vi "Sys config window-Get set control values.vi"(8 "error in (no error)":errorcluster, 11 "Function":T31) -> (0 "error out":errorcluster, 3 "output cluster":T1={"Triggers output setup"=[], "General trigger settings"={"Trigger 1 function"=enum."Encoder trigger", "Triggers loop clock (MHz)"=80.0}, "Calibration settings"={"Pockels cal.Zoom"=0, "Pockels cal.Dwell time (µs)"=0.0}, "Hardware Configuration"={"Dev. PC"=FALSE, "Swap XY on stage"=FALSE, "No of AOD"=0, "Computer MAC address"="", "Externalise Triggers"=FALSE, "Trigger HW config"={"Available Device List"=0, "Device Address"=""}, "DAQmx Chan"={"Pockels AO"="", "Hard shutter AO"="", "PMT AOs"="", "Galvo AOs"="", "Power meter AI"=""}, "XY stage available"=FALSE, "XY Stage"={"COM port"="", "Baudrate"=0, "Type"=""}, "Z stage available"=FALSE, "Z Stage config cluster"={"COM port"="COM7", "Baudrate"=0, "Type"=""}, "Encoder available"=FALSE, "Encoder"={"IP address"="224.0.1.103", "Port"=7000, "Wheel radius (cm)"=16.0, "Encoder Trigger"=""}, "VidRec available"=FALSE, "Cam VidRec"={"DO flag-Video record"="", "DO flag-Trial start"=""}, "Laser Power Control HW config"={"Laser Power Control"="", "Laser Power Modulation Control"=enum."NI"}, "Laser 1 available"=FALSE, "Laser 1 config cluster"={"COM port"="COM7", "Baud Rate"=0, "Type"=""}, "Prechirper 1 available"=FALSE, "Prechirper 1 config cluster"={"Type"="", "Baud Rate"=0, "COM port"="COM7"}, "Control system.FPGA available?"=FALSE, "Control Sys. HW config"={"Control system.FPGA Type"=enum."Virtex 5", "Control system.Network adapter name"="", "Control system.MAC address"="", "Control system.Ethernet Port"=0, "Control system.Ethernet Port Opened"=FALSE}, "DAQ FPGA HW Config"={"FGPA Ref"=refnum, "Target"="RIO0", "input card type"=enum."AC Card"}}, "System Config"={"Laser wavelength (nm)"=920.0, "DAQ FPGA System"={"Clock Freq (MHz) "=200.0, "Samples Wait after Trigger"=5080, "AOD fill"=4900, "StartupDelay"=0, "Slip Cycle (clock cycles)"=600000, "Add Cycle"=TRUE}, "Control system"={"AOD 1 Amplitude"=0, "AOD 2 Amplitude"=0, "AOD 3 Amplitude"=0, "AOD 4 Amplitude"=0, "AOD 5 Amplitude"=0, "AOD 6 Amplitude"=0, "T0 (ns)"=0.0, "Ta (ns)"=0.0, "Data Time Interval (ns)"=0.0, "Ctrl FPGA Clock (MHz)"=240.0}}, "Calibration config."={"Current Objective"="", "Objective Settings"=[], "PreChirper Values Preset ?"=FALSE, "PreChirper Settings"=[], "PreChirper Constants"={"a 1"=0, "b 1"=0, "c 1"=0, "a 2"=0, "b 2"=0, "c 2"=0, "lmin"=0, "lmax"=0}}, "General Setup"={"Microscope ID"="003", "Microscope Type"="AOLM", "Revision Number"="1.0.0.0", "Advanced Imaging"=FALSE, "Error Logging"=FALSE, "Performance Monitoring"=FALSE, "Max Allowed Trial Length"=60.0, "Initial Scan Resolution"=512.0, "Initial Acceptance Angle"=5.0, "Initial Laser Wavelength"=900.0, "Initial Dwell Time"=900.0}, "AOD Settings - distilled"={"AOD 1 thickness (mm)"=8.0, "AOD 2 thickness (mm)"=8.0, "AOD 3 thickness (mm)"=8.0, "AOD 4 thickness (mm)"=8.0, "AOD 1-2 separation (mm)"=50.0, "AOD 2-3 separation (mm)"=50.0, "AOD 3-4 separation (mm)"=50.0, "AOD 1 Centre (mm)"=7.5, "AOD 2 Centre (mm)"=7.5, "AOD 3 Centre (mm)"=7.5, "AOD 4 Centre (mm)"=7.5, "AOD 1 X Offset"=0.0, "AOD 2 X Offset"=0.0023, "AOD 3 X Offset"=0.0046, "AOD 4 X Offset"=0.0046, "AOD 1 Y Offset"=0.0, "AOD 2 Y Offset"=0.0, "AOD 3 Y Offset"=0.0023, "AOD 4 Y Offset"=0.0046, "Timing Offset AOD 1"=0.0, "Timing Offset AOD 2"=0.0, "Timing Offset AOD 3"=0.0, "Timing Offset AOD 4"=0.0, "AOL centre wavelength (nm)"=1.0, "AOL centre frequency (MHz)"=1.0, "Pair deflection ratio"=1.0, "AOL aperture (mm)"=15.0, "AOD fill time (us)"=1.0, "Diffraction mode"=1.0, "Crystal length (mm)"=0.0, "Acoustic velocity (m/s)"=1.0, "AOD Ord. Refractive index"=2.22}} {"System Config"."Control system"."Ctrl FPGA Clock (MHz)" min=80.0 max=500.0 step=1.0; "System Config"."Control system"."Data Time Interval (ns)" min=0.0 max=2048.0 step=1.0; "System Config"."Control system"."Ta (ns)" min=0.0 max=2048.0 step=1.0; "System Config"."Control system"."T0 (ns)" min=0.0 max=2048.0 step=1.0; "System Config"."Control system"."AOD 6 Amplitude" min=0 max=2048 step=1; "System Config"."Control system"."AOD 5 Amplitude" min=0 max=2048 step=1; "System Config"."Control system"."AOD 4 Amplitude" min=0 max=2048 step=1; "System Config"."Control system"."AOD 3 Amplitude" min=0 max=2048 step=1; "System Config"."Control system"."AOD 2 Amplitude" min=0 max=2048 step=1; "System Config"."Control system"."AOD 1 Amplitude" min=0 max=2048 step=1; "System Config"."Laser wavelength (nm)" min=800.0 max=1080.0 step=1.0; "Hardware Configuration"."Encoder"."Wheel radius (cm)" format="%#_13g"; "General trigger settings"."Triggers loop clock (MHz)" format="%#_13g"; "Triggers output setup"."Pulse width (us)" min=10 max=5000 step=1 format="%.0fµs"})   [LabVIEW 2017]
uses:
  Visualisation/Functional Imaging Viewer/Typedefs/Get-Set-Clear Control.ctl
  Configuration code/Typedefs/Initial config.ctl
  Peripherals Control/Triggers/Typedefs/Triggers output setup.ctl
  Peripherals Control/Triggers/Typedefs/Trigger setup element cluster.ctl
  Peripherals Control/Triggers/Typedefs/General trigger settings cluster.ctl
  Typedefs/Trigger 1 selector enum.ctl
  Configuration code/Typedefs/Pockels Calibration settings cluster.ctl
  Typedefs/Hardware Configuration settings.ctl
  Typedefs/Triggers HW config.ctl
  Typedefs/DAQmx physical channels cluster.ctl
  Typedefs/XY Stage config cluster.ctl
  Typedefs/Z Stage config cluster.ctl
  Typedefs/Encoder config cluster.ctl
  Typedefs/Cam VidRec HW config setup cluster.ctl
  Typedefs/Laser Power Control HW config.ctl
  Typedefs/Laser 1 config cluster.ctl
  Typedefs/PreChirper 1 config cluster.ctl
  Typedefs/Control Sys HW config cluster.ctl
  Typedefs/DAQ FPGA HW config cluster.ctl
  RIG-SPECIFIC FILES/FPGA Refs/FPGA Ref.ctl
  <vilib>/userdefined/High Color/nirio_resource_hc.ctl
  Typedefs/FPGA input type AC-DC.ctl
  Typedefs/System Configuration.ctl
  Typedefs/DAQ FPGA system config.ctl
  Typedefs/CTRL system config.ctl
  Typedefs/Calibration config.ctl
  Typedefs/Objective Config.ctl
  Typedefs/Prechirper Cal Config.ctl
  Typedefs/PreChirper constants.ctl
  Typedefs/General Setup.ctl
  Typedefs/AOD Settings-distilled.ctl
  Typedefs/HW config states enum.ctl
  Typedefs/fgv_actions.ctl
  Globals/Sys Config window globals.vi
  Global Variables/General Globals.vi
  Configuration code/Calibration/Globals/gl_Calibration globals.vi
panel:
  # "Thickness (mm)"
  # "X Offset"
  # "Separation (mm)"
  # "Y Offset"
  # "Centre (mm)"
  # "Timing Offset"
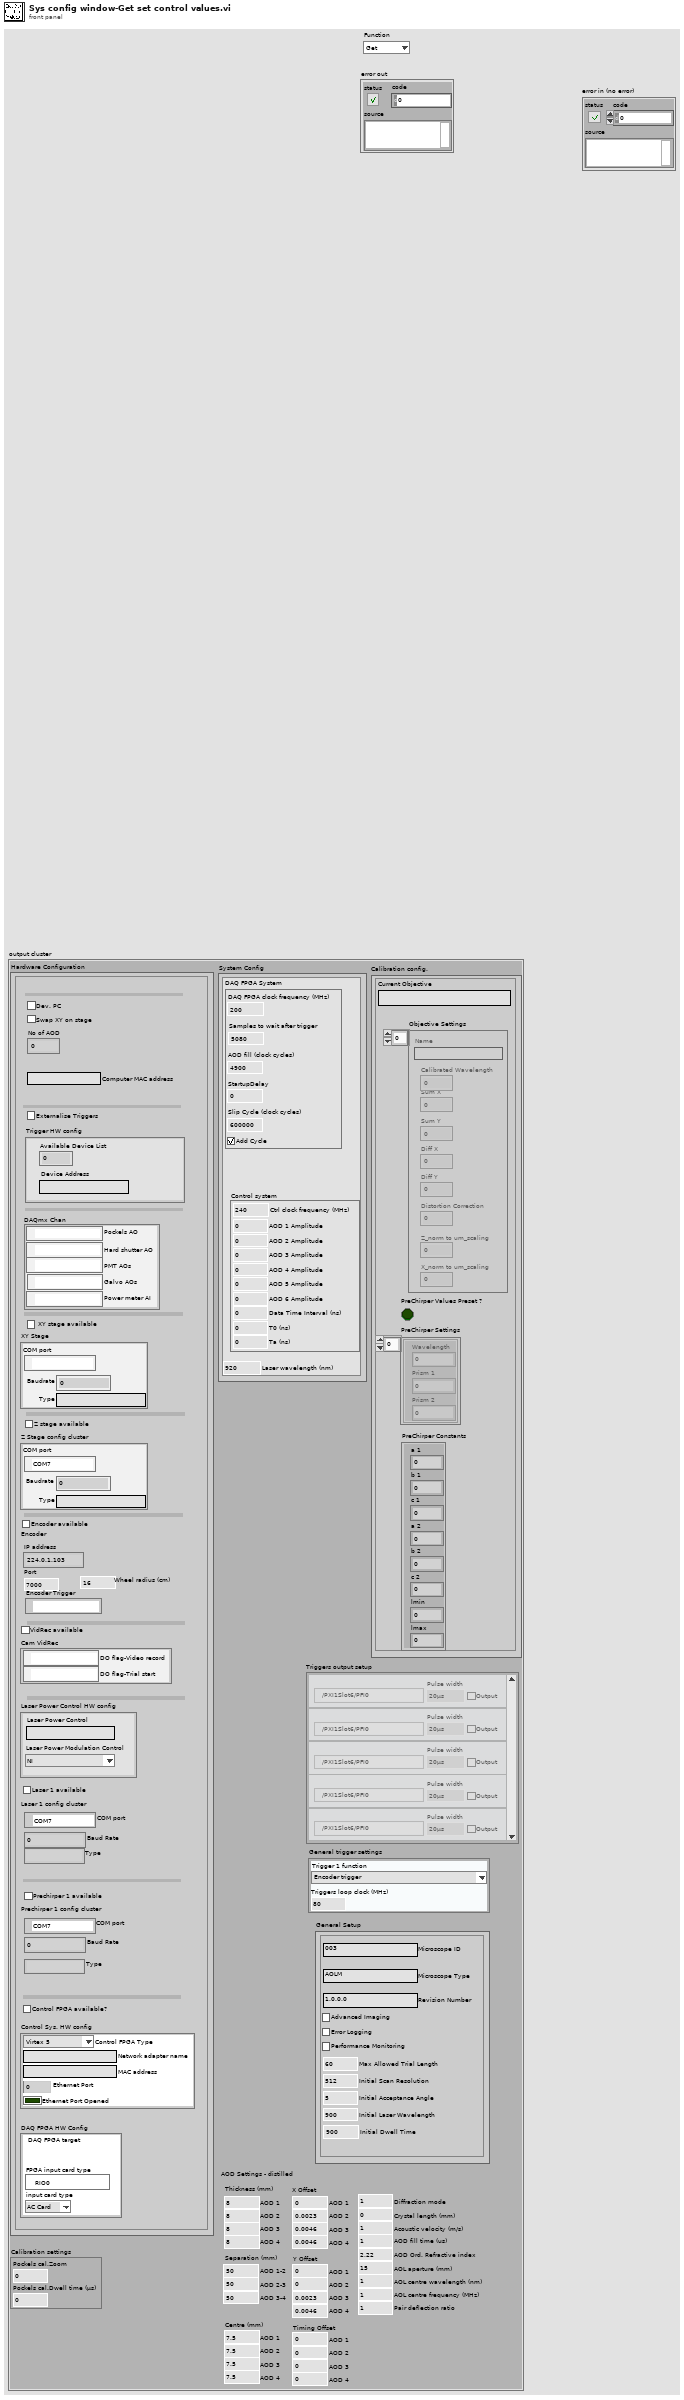
[diagram p1: front panel]
types:
  T1 = typedef "Initial config.ctl" = cluster{"Triggers output setup":T2, "General trigger settings":T4, "Calibration settings":T6, "Hardware Configuration":T7, "System Config":T22, "Calibration config.":T25, "General Setup":T29, "AOD Settings - distilled":T30}
  T2 = typedef "Triggers output setup.ctl" = T3[]
  T3 = typedef "Trigger setup element cluster.ctl" = cluster{"Name":string, "Output?":bool, "Output terminal":tag, "PXI backplane line":tag, "Pulse width (us)":u16}
  T4 = typedef "General trigger settings cluster.ctl" = cluster{"Trigger 1 function":T5, "Triggers loop clock (MHz)":dbl}
  T5 = typedef "Trigger 1 selector enum.ctl" = enum16{"Encoder trigger", "Line trigger", "Control system's ref frame acknowledgement"}
  T6 = typedef "Pockels Calibration settings cluster.ctl" = cluster{"Pockels cal.Zoom":u8, "Pockels cal.Dwell time (µs)":dbl}
  T7 = typedef "Hardware Configuration settings.ctl" = cluster{"Dev. PC":bool, "Swap XY on stage":bool, "No of AOD":u8, "Computer MAC address":string, "Externalise Triggers":bool, "Trigger HW config":T8, "DAQmx Chan":T9, "XY stage available":bool, "XY Stage":T10, "Z stage available":bool, "Z Stage config cluster":T11, "Encoder available":bool, "Encoder":T12, "VidRec available":bool, "Cam VidRec":T13, "Laser Power Control HW config":T14, "Laser 1 available":bool, "Laser 1 config cluster":T15, "Prechirper 1 available":bool, "Prechirper 1 config cluster":T16, "Control system.FPGA available?":bool, "Control Sys. HW config":T17, "DAQ FPGA HW Config":T18}
  T8 = typedef "Triggers HW config.ctl" = cluster{"Available Device List":i32, "Device Address":string}
  T9 = typedef "DAQmx physical channels cluster.ctl" = cluster{"Pockels AO":tag, "Hard shutter AO":tag, "PMT AOs":tag, "Galvo AOs":tag, "Power meter AI":tag}
  T10 = typedef "XY Stage config cluster.ctl" = cluster{"COM port":refnum<visa-resource-name>, "Baudrate":i32, "Type":string}
  T11 = typedef "Z Stage config cluster.ctl" = cluster{"COM port":refnum<visa-resource-name>, "Baudrate":i32, "Type":string}
  T12 = typedef "Encoder config cluster.ctl" = cluster{"IP address":string, "Port":u16, "Wheel radius (cm)":dbl, "Encoder Trigger":tag}
  T13 = typedef "Cam VidRec HW config setup cluster.ctl" = cluster{"DO flag-Video record":tag, "DO flag-Trial start":tag}
  T14 = typedef "Laser Power Control HW config.ctl" = cluster{"Laser Power Control":string, "Laser Power Modulation Control":enum16{"NI", "FPGA"}}
  T15 = typedef "Laser 1 config cluster.ctl" = cluster{"COM port":refnum<visa-resource-name>, "Baud Rate":i32, "Type":string}
  T16 = typedef "PreChirper 1 config cluster.ctl" = cluster{"Type":string, "Baud Rate":i32, "COM port":refnum<visa-resource-name>}
  T17 = typedef "Control Sys HW config cluster.ctl" = cluster{"Control system.FPGA Type":enum16{"Virtex 5", "Virtex 7"}, "Control system.Network adapter name":string, "Control system.MAC address":string, "Control system.Ethernet Port":u32, "Control system.Ethernet Port Opened":bool}
  T18 = typedef "DAQ FPGA HW config cluster.ctl" = cluster{"FGPA Ref":T19, "Target":T20, "input card type":T21}
  T19 = typedef "FPGA Ref.ctl" = refnum<k20>
  T20 = typedef "nirio_resource_hc.ctl" = tag
  T21 = typedef "FPGA input type AC-DC.ctl" = enum16{"AC Card", "DC Card"}
  T22 = typedef "System Configuration.ctl" = cluster{"Laser wavelength (nm)":dbl, "DAQ FPGA System":T23, "Control system":T24}
  T23 = typedef "DAQ FPGA system config.ctl" = cluster{"Clock Freq (MHz) ":dbl, "Samples Wait after Trigger":u16, "AOD fill":u16, "StartupDelay":i32, "Slip Cycle (clock cycles)":u32, "Add Cycle":bool}
  T24 = typedef "CTRL system config.ctl" = cluster{"AOD 1 Amplitude":i16, "AOD 2 Amplitude":i16, "AOD 3 Amplitude":i16, "AOD 4 Amplitude":i16, "AOD 5 Amplitude":i16, "AOD 6 Amplitude":i16, "T0 (ns)":dbl, "Ta (ns)":dbl, "Data Time Interval (ns)":dbl, "Ctrl FPGA Clock (MHz)":dbl}
  T25 = typedef "Calibration config.ctl" = cluster{"Current Objective":string, "Objective Settings":T26[], "PreChirper Values Preset ?":bool, "PreChirper Settings":T27[], "PreChirper Constants":T28}
  T26 = typedef "Objective Config.ctl" = cluster{"Name":string, "Sum X":dbl, "Sum Y":dbl, "Diff X":dbl, "Diff Y":dbl, "Distortion Correction":dbl, "Z_norm to um_scaling":dbl, "X_norm to um_scaling":dbl, "Calibrated Wavelength":dbl}
  T27 = typedef "Prechirper Cal Config.ctl" = cluster{"Wavelength":i32, "Prism 1":i32, "Prism 2":i32}
  T28 = typedef "PreChirper constants.ctl" = cluster{"a 1":i32, "b 1":i32, "c 1":i32, "a 2":i32, "b 2":i32, "c 2":i32, "lmin":i32, "lmax":i32}
  T29 = typedef "General Setup.ctl" = cluster{"Microscope ID":string, "Microscope Type":string, "Revision Number":string, "Advanced Imaging":bool, "Error Logging":bool, "Performance Monitoring":bool, "Max Allowed Trial Length":dbl, "Initial Scan Resolution":dbl, "Initial Acceptance Angle":dbl, "Initial Laser Wavelength":dbl, "Initial Dwell Time":dbl}
  T30 = typedef "AOD Settings-distilled.ctl" = cluster{"AOD 1 thickness (mm)":dbl, "AOD 2 thickness (mm)":dbl, "AOD 3 thickness (mm)":dbl, "AOD 4 thickness (mm)":dbl, "AOD 1-2 separation (mm)":dbl, "AOD 2-3 separation (mm)":dbl, "AOD 3-4 separation (mm)":dbl, "AOD 1 Centre (mm)":dbl, "AOD 2 Centre (mm)":dbl, "AOD 3 Centre (mm)":dbl, "AOD 4 Centre (mm)":dbl, "AOD 1 X Offset":dbl, "AOD 2 X Offset":dbl, "AOD 3 X Offset":dbl, "AOD 4 X Offset":dbl, "AOD 1 Y Offset":dbl, "AOD 2 Y Offset":dbl, "AOD 3 Y Offset":dbl, "AOD 4 Y Offset":dbl, "Timing Offset AOD 1":dbl, "Timing Offset AOD 2":dbl, "Timing Offset AOD 3":dbl, "Timing Offset AOD 4":dbl, "AOL centre wavelength (nm)":dbl, "AOL centre frequency (MHz)":dbl, "Pair deflection ratio":dbl, "AOL aperture (mm)":dbl, "AOD fill time (us)":dbl, "Diffraction mode":dbl, "Crystal length (mm)":dbl, "Acoustic velocity (m/s)":dbl, "AOD Ord. Refractive index":dbl}
  T31 = typedef "Get-Set-Clear Control.ctl" = enum16{"Get", "Set", "Clear"}
  T32 = enum16{"Initialise", "Load from file", "Save to file", "Read", "Write"}
  T33 = typedef "HW config states enum.ctl" = enum16{"Load from file", "Save to file", "Write all", "Read all", "Write XY stage settings", "Write DAQ FPGA settings", "Write Control FPGA settings", "Write Phys Channels", "Write System Config", "Write HW Config", "Save System Config", "Save HW Config", "Clear", "Compare from file"}
  T34 = typedef "HW config window refs cluster.ctl" = cluster{"VI's reference":refnum<vi>, "menu reference":refnum<k9>, "Pane":refnum<vi>, "Config Tab Control":refnum<vi>, "Triggers sub-tab control":refnum<vi>, "Microscope ID":refnum<vi>, "Microscope Type":refnum<vi>, "Revision Number":refnum<vi>, "Advanced Imaging":refnum<vi>, "Max Allowed Trial Length":refnum<vi>, "Initial Scan Resolution":refnum<vi>, "Initial Acceptance Angle":refnum<vi>, "Initial Laser Wavelength [nm] ":refnum<vi>, "Initial Dwell Time [us]":refnum<vi>, "Error Logging":refnum<vi>, "Performance Monitoring":refnum<vi>, "Ctrl FPGA available":refnum<vi>, "Control HW config":refnum<vi>, "Control System Config":refnum<vi>, "General trigger settings":refnum<vi>, "Trigger HW config":refnum<vi>, "Externalise Triggers":refnum<vi>, "[Triggers output setup]":refnum<vi>, "DAQ FPGA HW Config":refnum<vi>, "DAQ FPGA System Config":refnum<vi>, "Pockels AO":refnum<vi>, "Hard shutter AO":refnum<vi>, "PMT AOs":refnum<vi>, "Galvo AO":refnum<vi>, "Power meter AI":refnum<vi>, "XY stage available":refnum<vi>, "XY Stage config cluster":refnum<vi>, "Z stage available":refnum<vi>, "Z Stage config cluster":refnum<vi>, "Encoder available":refnum<vi>, "Encoder":refnum<vi>, "Encoder IP address":refnum<vi>, "Encoder port":refnum<vi>, "Wheel radius (cm)":refnum<vi>, "Demo mode":refnum<vi>, "Swap XY on stage":refnum<vi>, "Number of AODs":refnum<vi>, "Computer MAC add.":refnum<vi>, "Cam VidRec available":refnum<vi>, "Cam VidRec":refnum<vi>, "DO flag-Video record":refnum<vi>, "DO flag-Trial start":refnum<vi>, "AOD Settings (distilled)":refnum<vi>, "Pockels cal.Dwell time (µs)":refnum<vi>, "Pockels cal.Zoom":refnum<vi>, "Current Objective":refnum<vi>, "[Obj. Calib. Settings]":refnum<vi>, "Laser Wavelength":refnum<vi>, "Laser Power Control \nHW config":refnum<vi>, "Laser 1 available":refnum<vi>, "Laser 1 config":refnum<vi>, "Prechirper 1 available":refnum<vi>, "Prechirper 1 config":refnum<vi>, "PreChirp Preset Values":refnum<vi>, "[PreChirper Preset \nCalibration Values]":refnum<vi>, "Prechirper Constants":refnum<vi>}
  T35 = typedef "fgv_actions.ctl" = enum16{"Get", "Set"}
  T36 = typedef "AOL Properties Cluster.ctl" = cluster{"AOD 1 thickness (mm)":dbl, "AOD 2 thickness (mm)":dbl, "AOD 3 thickness (mm)":dbl, "AOD 4 thickness (mm)":dbl, "AOD 5 thickness (mm)":dbl, "AOD 6 thickness (mm)":dbl, "AOD 1-2 separation (mm)":dbl, "AOD 2-3 separation (mm)":dbl, "AOD 3-4 separation (mm)":dbl, "AOD 4-5 separation (mm)":dbl, "AOD 5-6 separation (mm)":dbl, "AOD 1 X Offset":dbl, "AOD 2 X Offset":dbl, "AOD 3 X Offset":dbl, "AOD 4 X Offset":dbl, "AOD 1 Y Offset":dbl, "AOD 2 Y Offset":dbl, "AOD 3 Y Offset":dbl, "AOD 4 Y Offset":dbl, "AOD 1 X Direction":dbl, "AOD 2 X Direction":dbl, "AOD 3 X Direction":dbl, "AOD 4 X Direction":dbl, "AOD 1 Y Direction":dbl, "AOD 2 Y Direction":dbl, "AOD 3 Y Direction":dbl, "AOD 4 Y Direction":dbl, "AOD 1 Centre (mm)":dbl, "AOD 2 Centre (mm)":dbl, "AOD 3 Centre (mm)":dbl, "AOD 4 Centre (mm)":dbl, "Timing Offset AOD 1":dbl, "Timing Offset AOD 2":dbl, "Timing Offset AOD 3":dbl, "Timing Offset AOD 4":dbl, "AOD Optical offset 1":dbl, "AOD Optical offset 2":dbl, "AOL aperture (mm)":dbl, "AOL centre wavelength (nm)":dbl, "AOL centre frequency (MHz)":dbl, "Diffraction mode":dbl, "Crystal length (mm)":dbl, "Acoustic velocity (m/s)":dbl, "Pair deflection ratio":dbl, "AOD fill time (us)":dbl, "AOD Ord. Refractive index":dbl, "AOD ExtraOrd. Refractive index":dbl}
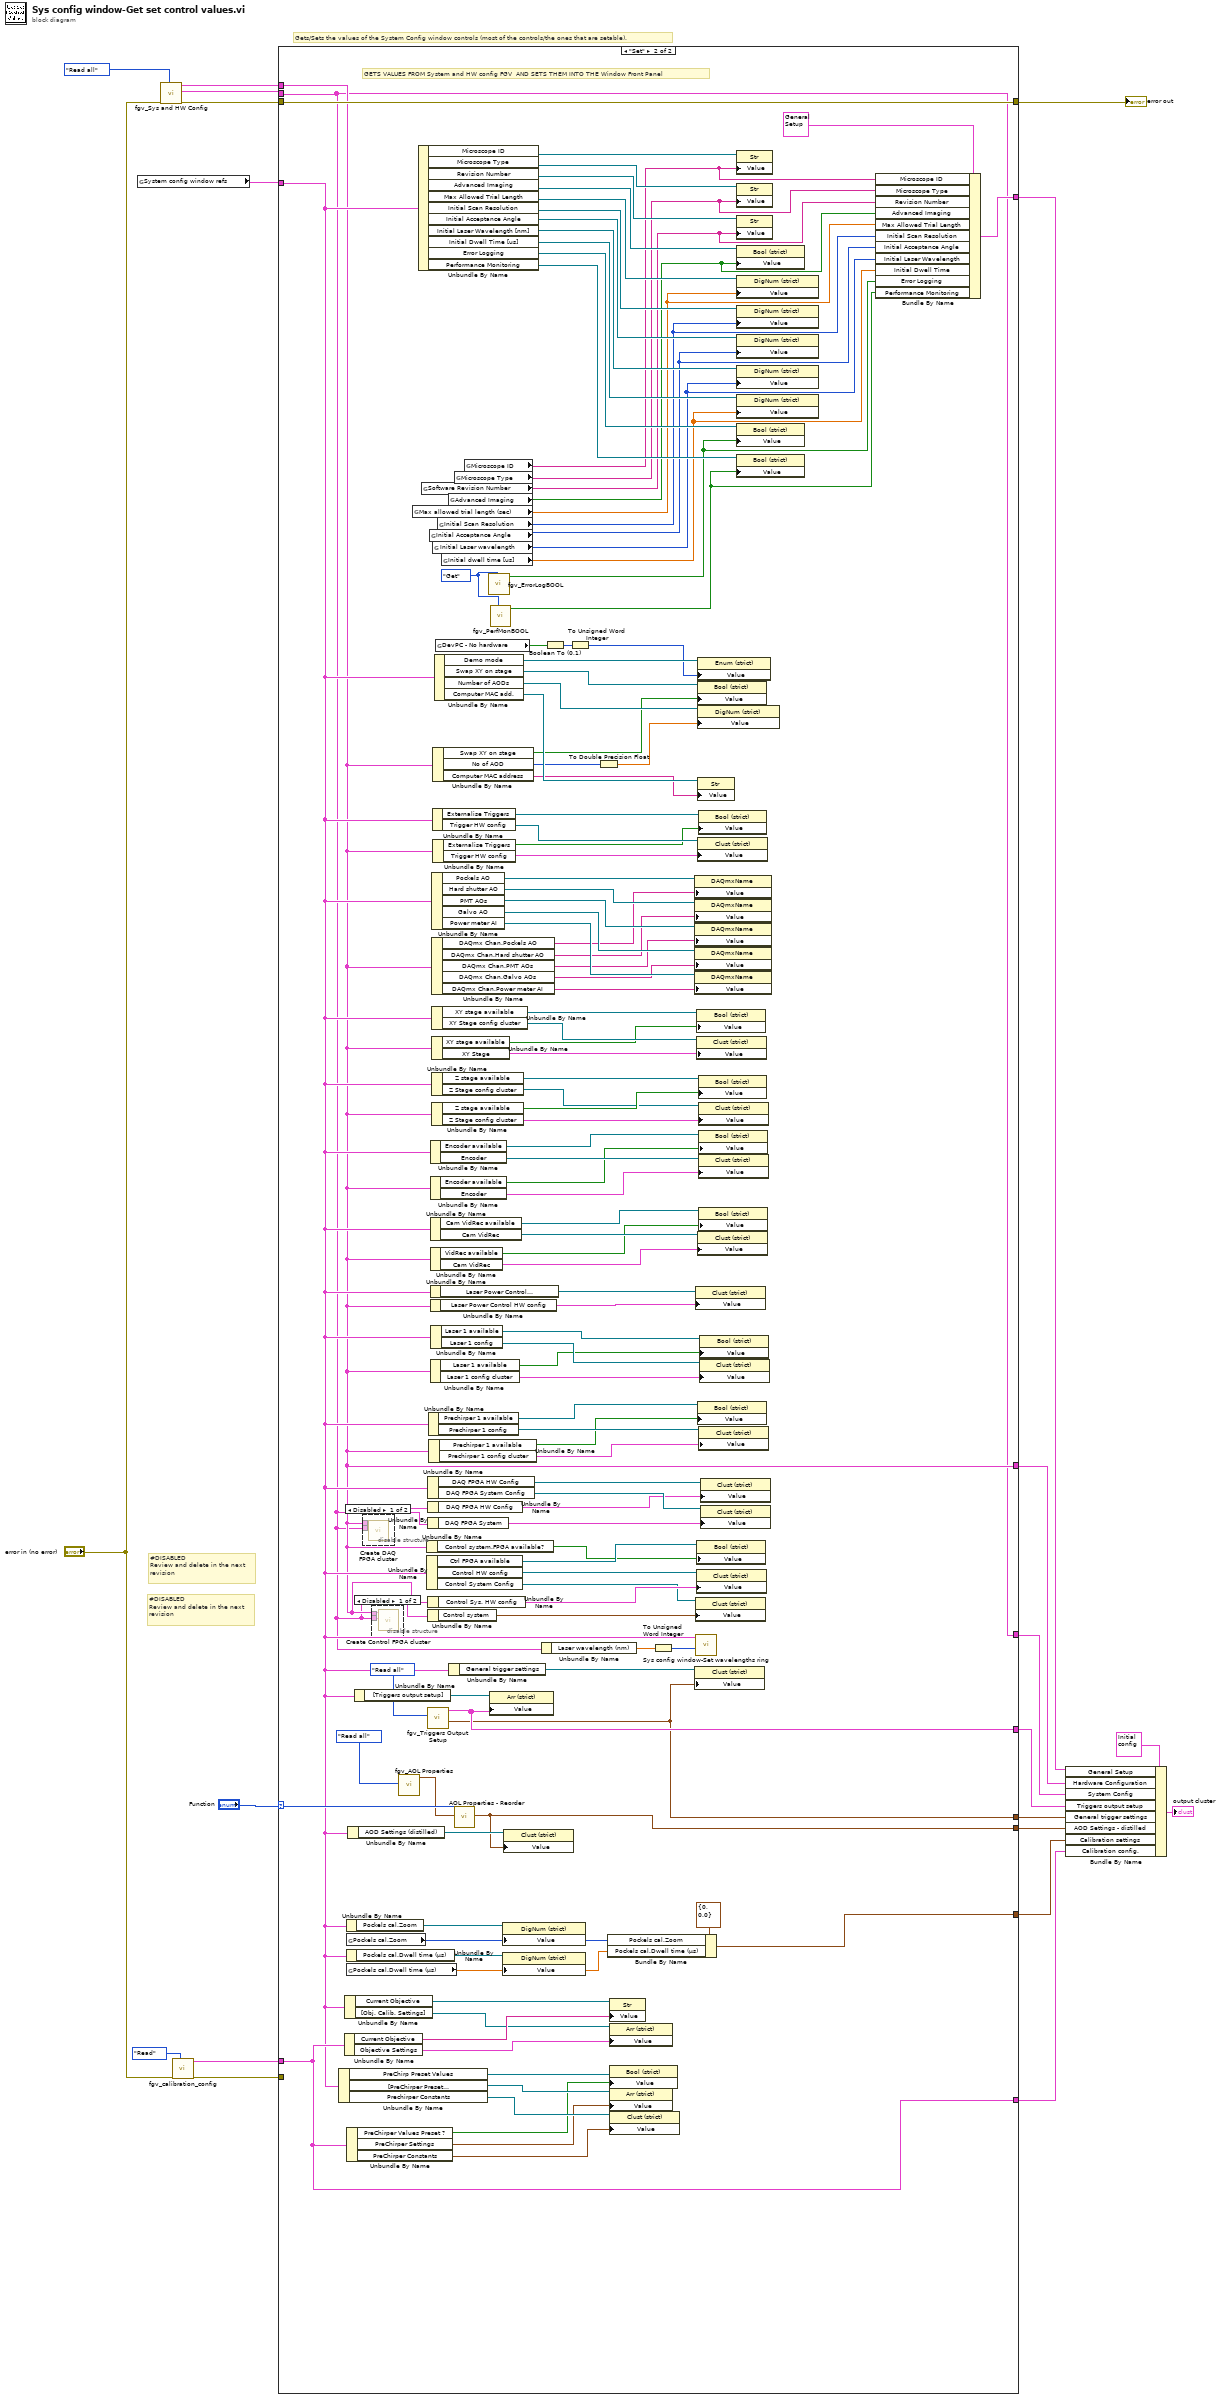
[diagram p0: block diagram]
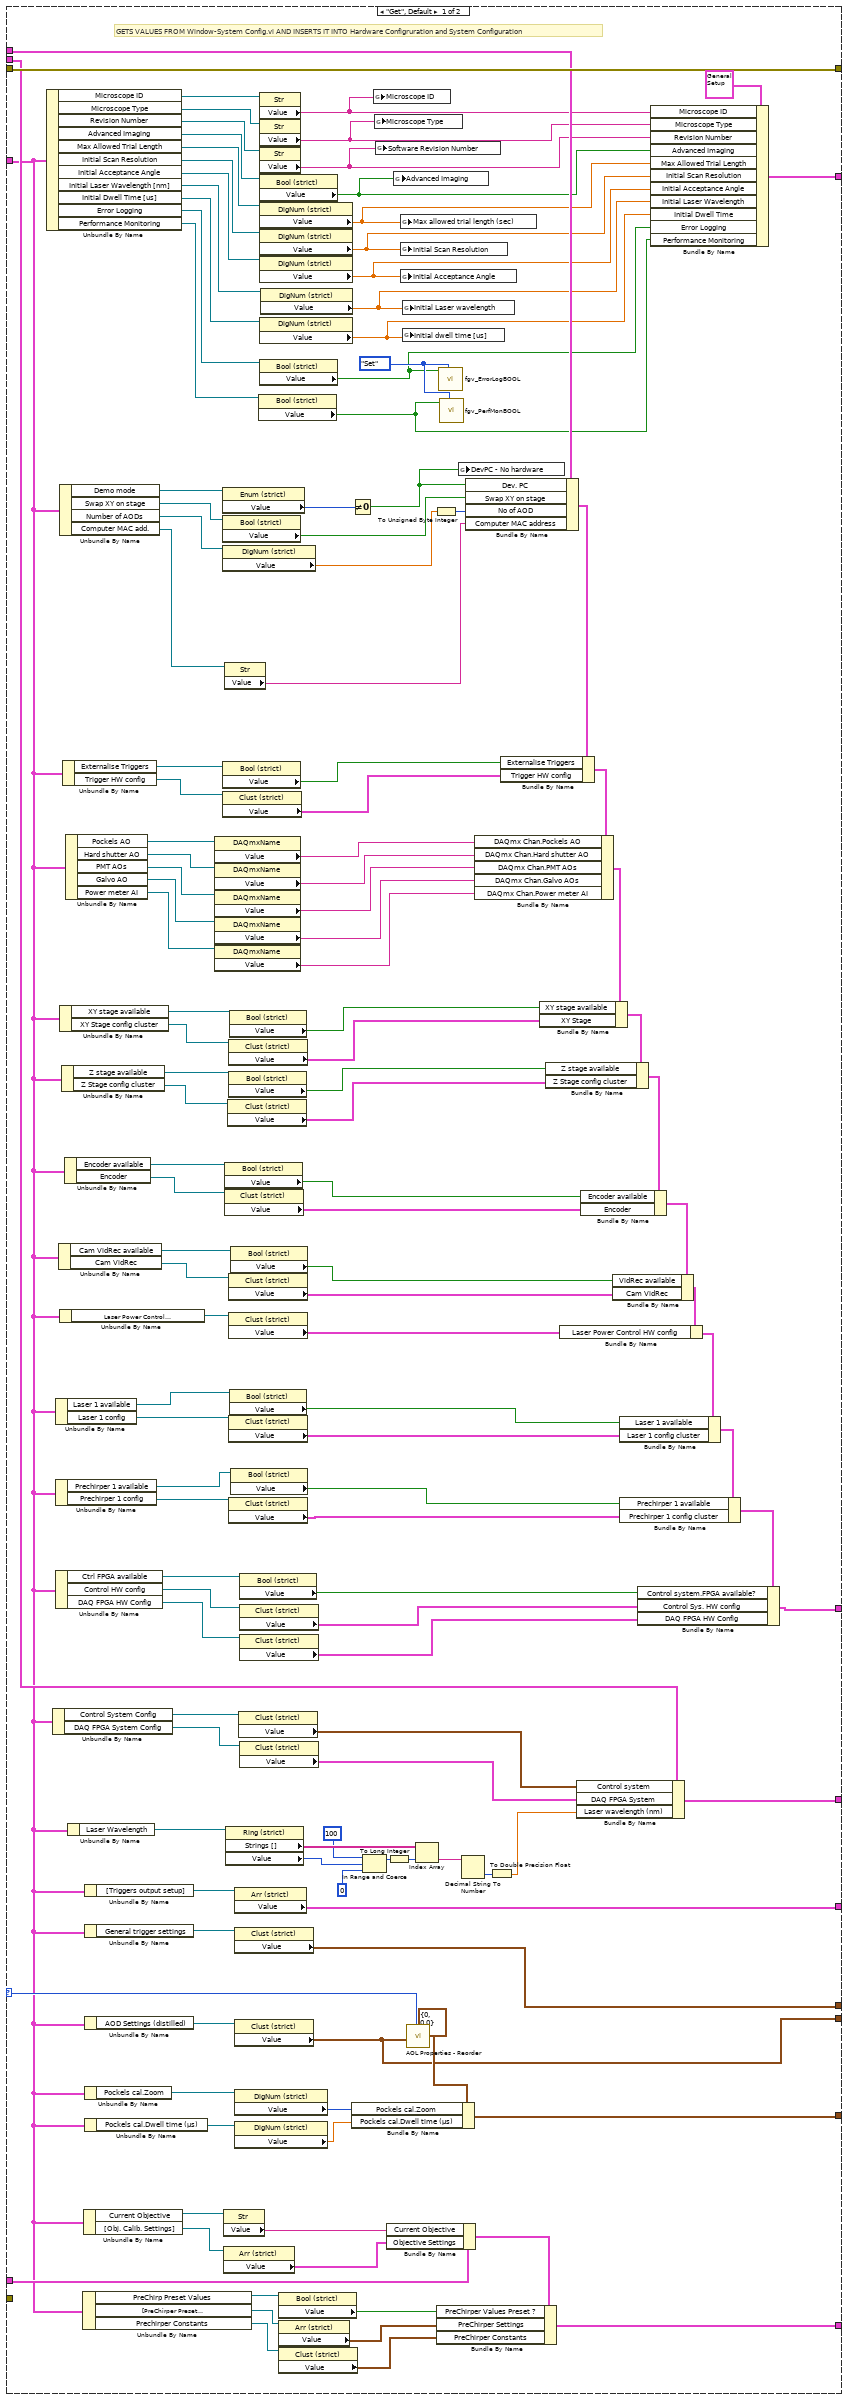
[diagram p2: hidden frame]
diagram:
  # "#DISABLED\nReview and delete in the next \nrevision"
  # "#DISABLED\nReview and delete in the next \nrevision"
  # "Gets/Sets the values of the System Config window controls (most of the controls/the ones that are setable)."
  n1 = global read "Sys Config window globals.vi" "System config window refs"() -> (w21:T34)
  n2 = call "fgv_Sys and HW Config.vi"("Function"=HW_config_states_enum."Read all", "error in (no error)"="error in (no error)") -> ("error out"=w16:errorcluster, "System Config OUT"=w13:T22, "Hardware Configuration OUT"=w17:T7)  [unwired: 7 in]
  n3 = call "fgv_calibration_config.vi"("Cal config ops"=T32."Read", "error in (no error)"="error in (no error)") -> ("error out"=w7:errorcluster, "Config cluster OUT"=w8:T25)  [unwired: 8 in]
  n4 = case shown="\"Set\"" "Function" {
    selector: "Function" -> [w67 w216]
    tunnel: w21 -> [w26 w187]
    tunnel: [w158 w162] -> w6
    tunnel: [w155 w268] -> w19
    tunnel: [w82 w270] -> w18
    tunnel: w17 -> [w50 w162]
    tunnel: w16 -> [w155 w268]
    tunnel: [w150 w262] -> w15
    tunnel: [w138 w258] -> w14
    tunnel: w13 -> [w84 w160]
    tunnel: w8 -> [w81 w207]
    tunnel: w7 -> [_ _]
    tunnel: [w83 w160] -> w5
    tunnel: [w69 w207] -> w4
    tunnel: [w32 w168] -> w3
    tunnel: [w31 w167] -> w2
    frame "Get", Default {
      w47 = fgv_actions."Set" ("FGV Actions")
      # "GETS VALUES FROM Window-System Config.vi AND INSERTS IT INTO Hardware Configruration and System Configuration"
      n5 = Unbundle By Name(w26) -> ("Microscope ID"=w137:refnum<vi>, "Microscope Type"=w136:refnum<vi>, "Revision Number"=w135:refnum<vi>, "Advanced Imaging"=w134:refnum<vi>, "Max Allowed Trial Length"=w133:refnum<vi>, "Initial Scan Resolution"=w132:refnum<vi>, "Initial Acceptance Angle"=w131:refnum<vi>, "Initial Laser Wavelength [nm]"=w49:refnum<vi>, "Initial Dwell Time [us]"=w48:refnum<vi>, "Error Logging"=w46:refnum<vi>, "Performance Monitoring"=w45:refnum<vi>)
      n6 = Unbundle By Name(w26) -> ("Control System Config"=w25:refnum<vi>, "DAQ FPGA System Config"=w23:refnum<vi>)
      n7 = Unbundle By Name(w26) -> ("Laser 1 available"=w54:refnum<vi>, "Laser 1 config"=w91:refnum<vi>)
      n8 = Unbundle By Name(w26) -> ("Prechirper 1 available"=w52:refnum<vi>, "Prechirper 1 config"=w87:refnum<vi>)
      n9 = Unbundle By Name(w26) -> ("Ctrl FPGA available"=w66:refnum<vi>, "Control HW config"=w30:refnum<vi>, "DAQ FPGA HW Config"=w28:refnum<vi>)
      n10 = Unbundle By Name(w26) -> ("Cam VidRec available"=w56:refnum<vi>, "Cam VidRec"=w98:refnum<vi>)
      n11 = Unbundle By Name(w26) -> ("Demo mode"=w130:refnum<vi>, "Swap XY on stage"=w129:refnum<vi>, "Number of AODs"=w128:refnum<vi>, "Computer MAC add."=w123:refnum<vi>)
      n12 = Unbundle By Name(w26) -> ("XY stage available"=w105:refnum<vi>, "XY Stage config cluster"=w104:refnum<vi>)
      n13 = Unbundle By Name(w26) -> ("Laser Power Control \nHW config"=w94:refnum<vi>)
      n14 = Unbundle By Name(w26) -> ("Z stage available"=w61:refnum<vi>, "Z Stage config cluster"=w62:refnum<vi>)
      n15 = Unbundle By Name(w26) -> ("Externalise Triggers"=w121:refnum<vi>, "Trigger HW config"=w120:refnum<vi>)
      n16 = Unbundle By Name(w26) -> ("Encoder available"=w59:refnum<vi>, "Encoder"=w100:refnum<vi>)
      n17 = Unbundle By Name(w26) -> ("Pockels AO"=w117:refnum<vi>, "Hard shutter AO"=w116:refnum<vi>, "PMT AOs"=w115:refnum<vi>, "Galvo AO"=w114:refnum<vi>, "Power meter AI"=w113:refnum<vi>)
      n18 = Unbundle By Name(w26) -> ("Laser Wavelength"=w149:refnum<vi>)
      n19 = Unbundle By Name(w26) -> ("PreChirp Preset Values"=w75:refnum<vi>, "[PreChirper Preset \nCalibration Values]"=w76:refnum<vi>, "Prechirper Constants"=w74:refnum<vi>)
      n20 = Unbundle By Name(w26) -> ("Current Objective"=w80:refnum<vi>, "[Obj. Calib. Settings]"=w78:refnum<vi>)
      n21 = Unbundle By Name(w26) -> ("[Triggers output setup]"=w157:refnum<vi>)
      n22 = Unbundle By Name(w26) -> ("General trigger settings"=w139:refnum<vi>)
      n23 = Unbundle By Name(w26) -> ("AOD Settings (distilled)"=w156:refnum<vi>)
      n24 = Unbundle By Name(w26) -> ("Pockels cal.Zoom"=w153:refnum<vi>)
      n25 = Unbundle By Name(w26) -> ("Pockels cal.Dwell time (µs)"=w154:refnum<vi>)
      n26 = property class="DAQmxName"(reference=w117) -> ("Value"=w112:string)  [unwired: 1 in, 2 out]
      n27 = property class="DAQmxName"(reference=w116) -> ("Value"=w111:string)  [unwired: 1 in, 2 out]
      n28 = property class="DAQmxName"(reference=w115) -> ("Value"=w110:string)  [unwired: 1 in, 2 out]
      n29 = property class="DAQmxName"(reference=w114) -> ("Value"=w109:string)  [unwired: 1 in, 2 out]
      n30 = property class="DAQmxName"(reference=w113) -> ("Value"=w108:string)  [unwired: 1 in, 2 out]
      n31 = property class="Enum (strict)"(reference=w130) -> ("Value"=w127:enum16{"Full functionality", "Demo mode"})  [unwired: 1 in, 2 out]
      n32 = property class="Bool (strict)"(reference=w129) -> ("Value"=w126:bool)  [unwired: 1 in, 2 out]
      n33 = property class="DigNum (strict)"(reference=w128) -> ("Value"=w124:dbl)  [unwired: 1 in, 2 out]
      n34 = property class="Bool (strict)"(reference=w121) -> ("Value"=w119:bool)  [unwired: 1 in, 2 out]
      n35 = property class="Clust (strict)"(reference=w120) -> ("Value"=w118:T8)  [unwired: 1 in, 2 out]
      n36 = property class="Str"(reference=w80) -> ("Value"=w79:string)  [unwired: 1 in, 2 out]
      n37 = property class="Arr (strict)"(reference=w78) -> ("Value"=w77:T26[])  [unwired: 1 in, 2 out]
      n38 = property class="Str"(reference=w123) -> ("Value"=w122:string)  [unwired: 1 in, 2 out]
      n39 = property class="Clust (strict)"(reference=w100) -> ("Value"=w99:T12)  [unwired: 1 in, 2 out]
      n40 = property class="Bool (strict)"(reference=w59) -> ("Value"=w57:bool)  [unwired: 1 in, 2 out]
      n41 = property on="Property Node" class="Ring (strict)"(reference=w149) -> ("Strings []"=w148:string[], "Value"=w145:u16)  [unwired: 1 in, 2 out]
      n42 = property class="Clust (strict)"(reference=w62) -> ("Value"=w64:T11)  [unwired: 1 in, 2 out]
      n43 = property class="Clust (strict)"(reference=w104) -> ("Value"=w101:T10)  [unwired: 1 in, 2 out]
      n44 = property class="Bool (strict)"(reference=w61) -> ("Value"=w63:bool)  [unwired: 1 in, 2 out]
      n45 = property class="Clust (strict)"(reference=w98) -> ("Value"=w97:T13)  [unwired: 1 in, 2 out]
      n46 = property class="Clust (strict)"(reference=w94) -> ("Value"=w92:T14)  [unwired: 1 in, 2 out]
      n47 = property class="Clust (strict)"(reference=w91) -> ("Value"=w90:T15)  [unwired: 1 in, 2 out]
      n48 = property class="Clust (strict)"(reference=w87) -> ("Value"=w88:T16)  [unwired: 1 in, 2 out]
      n49 = property class="Bool (strict)"(reference=w105) -> ("Value"=w102:bool)  [unwired: 1 in, 2 out]
      n50 = property class="Bool (strict)"(reference=w54) -> ("Value"=w53:bool)  [unwired: 1 in, 2 out]
      n51 = property class="Bool (strict)"(reference=w56) -> ("Value"=w55:bool)  [unwired: 1 in, 2 out]
      n52 = property class="Bool (strict)"(reference=w52) -> ("Value"=w51:bool)  [unwired: 1 in, 2 out]
      n53 = property class="Arr (strict)"(reference=w157) -> ("Value"=w82:T2)  [unwired: 1 in, 2 out]
      n54 = property class="Clust (strict)"(reference=w139) -> ("Value"=w138:T4)  [unwired: 1 in, 2 out]
      n55 = property class="Clust (strict)"(reference=w156) -> ("Value"=w31:T30)  [unwired: 1 in, 2 out]
      n56 = property class="DigNum (strict)"(reference=w153) -> ("Value"=w151:u8)  [unwired: 1 in, 2 out]
      n57 = property class="DigNum (strict)"(reference=w154) -> ("Value"=w152:dbl)  [unwired: 1 in, 2 out]
      n58 = property class="Clust (strict)"(reference=w25) -> ("Value"=w24:T24)  [unwired: 1 in, 2 out]
      n59 = property class="Bool (strict)"(reference=w66) -> ("Value"=w65:bool)  [unwired: 1 in, 2 out]
      n60 = property class="Clust (strict)"(reference=w30) -> ("Value"=w29:T17)  [unwired: 1 in, 2 out]
      n61 = property class="Clust (strict)"(reference=w28) -> ("Value"=w27:T18)  [unwired: 1 in, 2 out]
      n62 = property class="Clust (strict)"(reference=w23) -> ("Value"=w22:T23)  [unwired: 1 in, 2 out]
      n63 = property class="Bool (strict)"(reference=w45) -> ("Value"=w33:bool)  [unwired: 1 in, 2 out]
      n64 = property class="Str"(reference=w137) -> ("Value"=w43:string)  [unwired: 1 in, 2 out]
      n65 = property class="Str"(reference=w136) -> ("Value"=w42:string)  [unwired: 1 in, 2 out]
      n66 = property class="Str"(reference=w135) -> ("Value"=w41:string)  [unwired: 1 in, 2 out]
      n67 = property class="Bool (strict)"(reference=w134) -> ("Value"=w40:bool)  [unwired: 1 in, 2 out]
      n68 = property class="DigNum (strict)"(reference=w133) -> ("Value"=w39:dbl)  [unwired: 1 in, 2 out]
      n69 = property class="DigNum (strict)"(reference=w132) -> ("Value"=w38:dbl)  [unwired: 1 in, 2 out]
      n70 = property class="DigNum (strict)"(reference=w131) -> ("Value"=w37:dbl)  [unwired: 1 in, 2 out]
      n71 = property class="DigNum (strict)"(reference=w48) -> ("Value"=w35:dbl)  [unwired: 1 in, 2 out]
      n72 = property class="Bool (strict)"(reference=w46) -> ("Value"=w34:bool)  [unwired: 1 in, 2 out]
      n73 = property class="DigNum (strict)"(reference=w49) -> ("Value"=w36:dbl)  [unwired: 1 in, 2 out]
      n74 = property class="Bool (strict)"(reference=w75) -> ("Value"=w72:bool)  [unwired: 1 in, 2 out]
      n75 = property class="Arr (strict)"(reference=w76) -> ("Value"=w71:T27[])  [unwired: 1 in, 2 out]
      n76 = property class="Clust (strict)"(reference=w74) -> ("Value"=w70:T28)  [unwired: 1 in, 2 out]
      n77 = Not Equal To 0?(x=w127) -> (x != 0?=w95:bool)
      n78 = Bundle By Name(cluster=T6 {"Pockels cal.Zoom"=0, "Pockels cal.Dwell time (µs)"=0.0} ("Calibration settings"), "Pockels cal.Zoom"=w151, "Pockels cal.Dwell time (µs)"=w152) -> (w150:T6)
      n79 = In Range and Coerce(upper limit=u16 100, x=w145, lower limit=u16 0) -> (coerced(x)=w144:u16)  [unwired: 1 out]
      n80 = global write "General Globals.vi" "Microscope ID"(w43) -> ()
      n81 = global write "General Globals.vi" "Microscope Type"(w42) -> ()
      n82 = global write "General Globals.vi" "Software Revision Number"(w41) -> ()
      n83 = Bundle By Name(cluster=w81, "Current Objective"=w79, "Objective Settings"=w77) -> (w73:T25)
      n84 = To Long Integer(number=w144) -> (32bit integer=w143:i32)
      n85 = global write "General Globals.vi" "Advanced Imaging"(w40) -> ()
      n86 = global write "General Globals.vi" "Max allowed trial length (sec)"(w39) -> ()
      n87 = global write "General Globals.vi" "Initial Scan Resolution"(w38) -> ()
      n88 = global write "General Globals.vi" "Initial Acceptance Angle"(w37) -> ()
      n89 = global write "General Globals.vi" "Initial Laser wavelength"(w36) -> ()
      n90 = global write "General Globals.vi" "Initial dwell time [us]"(w35) -> ()
      n91 = call "AOL Properties - Reorder.vi"("Function"=w67, "Value"=w31) -> ()  [unwired: 8 in, 2 out]
      n92 = Index Array(array=w148, index=w143) -> (element=w141:string)
      n93 = To Unsigned Byte Integer(number=w124) -> (unsigned 8bit integer=w125:u8)
      n94 = Bundle By Name(cluster=w73, "PreChirper Values Preset ?"=w72, "PreChirper Settings"=w71, "PreChirper Constants"=w70) -> (w69:T25)
      n95 = call "fgv_ErrorLogBOOL.vi"("FGV Actions"=w47, "Error Logging ON [IN] ?"=w34) -> ()  [unwired: 8 in, 2 out]
      n96 = call "fgv_PerfMonBOOL.vi"("FGV Actions"=w47, "Perf Mon [IN]"=w33) -> ()  [unwired: 8 in, 2 out]
      n97 = global write "General Globals.vi" "DevPC - No hardware"(w95) -> ()
      n98 = Decimal String To Number(string=w141) -> (number=w140:i32)  [unwired: 2 in, 1 out]
      n99 = Bundle By Name(cluster=w50, "Dev. PC"=w95, "Swap XY on stage"=w126, "No of AOD"=w125, "Computer MAC address"=w122) -> (w107:T7)
      n100 = To Double Precision Float(number=w140) -> (double precision float=w68:dbl)
      n101 = Bundle By Name(cluster=w107, "Externalise Triggers"=w119, "Trigger HW config"=w118) -> (w106:T7)
      n102 = Bundle By Name(cluster=w106, "DAQmx Chan.Pockels AO"=w112, "DAQmx Chan.Hard shutter AO"=w111, "DAQmx Chan.PMT AOs"=w110, "DAQmx Chan.Galvo AOs"=w109, "DAQmx Chan.Power meter AI"=w108) -> (w103:T7)
      n103 = Bundle By Name(cluster=w103, "XY stage available"=w102, "XY Stage"=w101) -> (w60:T7)
      n104 = Bundle By Name(cluster=w60, "Z stage available"=w63, "Z Stage config cluster"=w64) -> (w58:T7)
      n105 = Bundle By Name(cluster=w84, "Control system"=w24, "DAQ FPGA System"=w22, "Laser wavelength (nm)"=w68) -> (w83:T22)
      n106 = Bundle By Name(cluster=w58, "Encoder available"=w57, "Encoder"=w99) -> (w96:T7)
      n107 = Bundle By Name(cluster=w96, "VidRec available"=w55, "Cam VidRec"=w97) -> (w93:T7)
      n108 = Bundle By Name(cluster=w93, "Laser Power Control HW config"=w92) -> (w89:T7)
      n109 = Bundle By Name(cluster=w89, "Laser 1 available"=w53, "Laser 1 config cluster"=w90) -> (w86:T7)
      n110 = Bundle By Name(cluster=w86, "Prechirper 1 available"=w51, "Prechirper 1 config cluster"=w88) -> (w85:T7)
      n111 = Bundle By Name(cluster=w85, "Control system.FPGA available?"=w65, "Control Sys. HW config"=w29, "DAQ FPGA HW Config"=w27) -> (w158:T7)
      n112 = Bundle By Name(cluster=T29 {"Microscope ID"="003", "Microscope Type"="AOLM", "Revision Number"="1.0.0.0", "Advanced Imaging"=FALSE, "Error Logging"=FALSE, "Performance Monitoring"=FALSE, "Max Allowed Trial Length"=60.0, "Initial Scan Resolution"=512.0, "Initial Acceptance Angle"=5.0, "Initial Laser Wavelength"=900.0, "Initial Dwell Time"=900.0} ("Cluster"), "Microscope ID"=w43, "Microscope Type"=w42, "Revision Number"=w41, "Advanced Imaging"=w40, "Max Allowed Trial Length"=w39, "Initial Scan Resolution"=w38, "Initial Acceptance Angle"=w37, "Initial Laser Wavelength"=w36, "Initial Dwell Time"=w35, "Error Logging"=w34, "Performance Monitoring"=w33) -> (w32:T29)
    }
    frame "Set" {
      w181 = fgv_actions."Get" ("FGV Actions")
      # "GETS VALUES FROM System and HW config FGV  AND SETS THEM INTO THE Window Front Panel"
      n113 = Unbundle By Name(w187) -> ("PreChirp Preset Values"=w206:refnum<vi>, "[PreChirper Preset \nCalibration Values]"=w205:refnum<vi>, "Prechirper Constants"=w204:refnum<vi>)
      n114 = Unbundle By Name(w207) -> ("Current Objective"=w210:string, "Objective Settings"=w208:T26[])
      n115 = Unbundle By Name(w187) -> ("Current Objective"=w211:refnum<vi>, "[Obj. Calib. Settings]"=w209:refnum<vi>)
      n116 = Unbundle By Name(w187) -> ("Pockels cal.Zoom"=w266:refnum<vi>)
      n117 = global read "gl_Calibration globals.vi" "Pockels cal.Zoom"() -> (w264:u8)
      n118 = Unbundle By Name(w187) -> ("Pockels cal.Dwell time (µs)"=w267:refnum<vi>)
      n119 = global read "gl_Calibration globals.vi" "Pockels cal.Dwell time (µs)"() -> (w263:dbl)
      n120 = Unbundle By Name(w207) -> ("PreChirper Values Preset ?"=w203:bool, "PreChirper Settings"=w202:T27[], "PreChirper Constants"=w201:T28)
      n121 = Unbundle By Name(w187) -> ("AOD Settings (distilled)"=w271:refnum<vi>)
      n122 = Unbundle By Name(w187) -> ("[Triggers output setup]"=w274:refnum<vi>)
      n123 = disable-structure shown="Disabled" {
        disable-tunnel: w162 -> [w279 _]
        disable-tunnel: w160 -> [w278 _]
        frame Disabled {
          n124 = call "Create DAQ FPGA cluster.vi"("System Config"=w278, "Hardware Configuration"=w279) -> ()  [unwired: 9 in, 1 out]
        }
        frame Enabled {
        }
      }
      n125 = disable-structure shown="Disabled" {
        disable-tunnel: w162 -> [w281 _]
        disable-tunnel: w160 -> [w280 _]
        frame Disabled {
          n126 = call "Create Control FPGA cluster.vi"("System Config"=w280, "Hardware Configuration"=w281) -> ()  [unwired: 9 in, 1 out]
        }
        frame Enabled {
        }
      }
      n127 = call "fgv_AOL Properties.vi"("Function"=HW_config_states_enum."Read all") -> ("AOL Properties out"=w215:T36)  [unwired: 9 in, 1 out]
      n128 = global read "General Globals.vi" "Max allowed trial length (sec)"() -> (w175:dbl)
      n129 = Unbundle By Name(w187) -> ("Microscope ID"=w257:refnum<vi>, "Microscope Type"=w256:refnum<vi>, "Revision Number"=w255:refnum<vi>, "Advanced Imaging"=w254:refnum<vi>, "Max Allowed Trial Length"=w253:refnum<vi>, "Initial Scan Resolution"=w252:refnum<vi>, "Initial Acceptance Angle"=w251:refnum<vi>, "Initial Laser Wavelength [nm]"=w185:refnum<vi>, "Initial Dwell Time [us]"=w184:refnum<vi>, "Error Logging"=w183:refnum<vi>, "Performance Monitoring"=w182:refnum<vi>)
      n130 = global read "General Globals.vi" "Software Revision Number"() -> (w177:string)
      n131 = Unbundle By Name(w162) -> ("Control system.FPGA available?"=w186:bool)
      n132 = Unbundle By Name(w187) -> ("Ctrl FPGA available"=w188:refnum<vi>, "Control HW config"=w269:refnum<vi>, "Control System Config"=w165:refnum<vi>)
      n133 = Unbundle By Name(w187) -> ("DAQ FPGA HW Config"=w276:refnum<vi>, "DAQ FPGA System Config"=w163:refnum<vi>)
      n134 = Unbundle By Name(w162) -> ("DAQ FPGA HW Config"=w161:T18)
      n135 = Unbundle By Name(w160) -> ("DAQ FPGA System"=w159:T23)
      n136 = Unbundle By Name(w162) -> ("Control Sys. HW config"=w166:T17)
      n137 = Unbundle By Name(w160) -> ("Control system"=w164:T24)
      n138 = call "fgv_Triggers Output Setup.vi"("Function"=HW_config_states_enum."Read all") -> ("General trigger settings"=w258:T4, "Triggers output setup"=w270:T2)  [unwired: 8 in, 1 out]
      n139 = Unbundle By Name(w187) -> ("Prechirper 1 available"=w190:refnum<vi>, "Prechirper 1 config"=w217:refnum<vi>)
      n140 = Unbundle By Name(w162) -> ("Prechirper 1 available"=w189:bool, "Prechirper 1 config cluster"=w218:T16)
      n141 = global read "General Globals.vi" "Initial Acceptance Angle"() -> (w173:i32)
      n142 = Unbundle By Name(w187) -> ("Encoder available"=w196:refnum<vi>, "Encoder"=w224:refnum<vi>)
      n143 = Unbundle By Name(w162) -> ("Encoder available"=w195:bool, "Encoder"=w223:T12)
      n144 = Unbundle By Name(w187) -> ("Cam VidRec available"=w194:refnum<vi>, "Cam VidRec"=w222:refnum<vi>)
      n145 = Unbundle By Name(w162) -> ("VidRec available"=w193:bool, "Cam VidRec"=w221:T13)
      n146 = Unbundle By Name(w187) -> ("Laser Power Control \nHW config"=w220:refnum<vi>)
      n147 = Unbundle By Name(w162) -> ("Laser Power Control HW config"=w219:T14)
      n148 = Unbundle By Name(w162) -> ("Laser 1 available"=w191:bool, "Laser 1 config cluster"=w275:T15)
      n149 = Unbundle By Name(w187) -> ("Laser 1 available"=w192:refnum<vi>, "Laser 1 config"=w277:refnum<vi>)
      n150 = Unbundle By Name(w187) -> ("Pockels AO"=w238:refnum<vi>, "Hard shutter AO"=w237:refnum<vi>, "PMT AOs"=w236:refnum<vi>, "Galvo AO"=w235:refnum<vi>, "Power meter AI"=w234:refnum<vi>)
      n151 = Unbundle By Name(w162) -> ("DAQmx Chan.Pockels AO"=w233:tag, "DAQmx Chan.Hard shutter AO"=w232:tag, "DAQmx Chan.PMT AOs"=w231:tag, "DAQmx Chan.Galvo AOs"=w230:tag, "DAQmx Chan.Power meter AI"=w229:tag)
      n152 = Unbundle By Name(w187) -> ("XY stage available"=w228:refnum<vi>, "XY Stage config cluster"=w227:refnum<vi>)
      n153 = Unbundle By Name(w162) -> ("XY stage available"=w226:bool, "XY Stage"=w225:T10)
      n154 = Unbundle By Name(w187) -> ("Z stage available"=w197:refnum<vi>, "Z Stage config cluster"=w198:refnum<vi>)
      n155 = Unbundle By Name(w162) -> ("Z stage available"=w199:bool, "Z Stage config cluster"=w200:T11)
      n156 = Unbundle By Name(w187) -> ("Externalise Triggers"=w242:refnum<vi>, "Trigger HW config"=w241:refnum<vi>)
      n157 = global read "General Globals.vi" "Initial Laser wavelength"() -> (w172:i32)
      n158 = Unbundle By Name(w162) -> ("Swap XY on stage"=w246:bool, "No of AOD"=w245:u8, "Computer MAC address"=w243:string)
      n159 = Unbundle By Name(w162) -> ("Externalise Triggers"=w240:bool, "Trigger HW config"=w239:T8)
      n160 = Unbundle By Name(w187) -> ("Demo mode"=w250:refnum<vi>, "Swap XY on stage"=w249:refnum<vi>, "Number of AODs"=w248:refnum<vi>, "Computer MAC add."=w247:refnum<vi>)
      n161 = global read "General Globals.vi" "DevPC - No hardware"() -> (w214:bool)
      n162 = global read "General Globals.vi" "Initial Scan Resolution"() -> (w174:i32)
      n163 = global read "General Globals.vi" "Initial dwell time [us]"() -> (w171:dbl)
      n164 = global read "General Globals.vi" "Advanced Imaging"() -> (w176:bool)
      n165 = Unbundle By Name(w187) -> ("General trigger settings"=w259:refnum<vi>)
      n166 = global read "General Globals.vi" "Microscope Type"() -> (w178:string)
      n167 = call "AOL Properties - Reorder.vi"("Function"=w216, "AOL Properties out"=w215) -> ("Value"=w167:T30)  [unwired: 8 in, 1 out]
      n168 = global read "General Globals.vi" "Microscope ID"() -> (w179:string)
      n169 = call "fgv_ErrorLogBOOL.vi"("FGV Actions"=w181) -> ("Error Logging ON [OUT]"=w170:bool)  [unwired: 9 in, 1 out]
      n170 = property class="Arr (strict)"(reference=w274, "Value"=w270) -> ()  [unwired: 1 in, 2 out]
      n171 = call "fgv_PerfMonBOOL.vi"("FGV Actions"=w181) -> ("Perf Mon [OUT]"=w169:bool)  [unwired: 9 in, 1 out]
      n172 = property class="DigNum (strict)"(reference=w266, "Value"=w264) -> ()  [unwired: 1 in, 2 out]
      n173 = property class="DigNum (strict)"(reference=w267, "Value"=w263) -> ()  [unwired: 1 in, 2 out]
      n174 = property class="Clust (strict)"(reference=w271, "Value"=w167) -> ()  [unwired: 1 in, 2 out]
      n175 = Unbundle By Name(w160) -> ("Laser wavelength (nm)"=w261:dbl)
      n176 = Boolean To (0,1)(Boolean=w214) -> (0, 1=w213:i16)
      n177 = To Unsigned Word Integer(number=w213) -> (unsigned 16bit integer=w212:u16)
      n178 = To Double Precision Float(number=w245) -> (double precision float=w244:dbl)
      n179 = Bundle By Name(cluster=T6 {"Pockels cal.Zoom"=0, "Pockels cal.Dwell time (µs)"=0.0} ("Calibration settings"), "Pockels cal.Zoom"=w264, "Pockels cal.Dwell time (µs)"=w263) -> (w262:T6)
      n180 = property class="Str"(reference=w211, "Value"=w210) -> ()  [unwired: 1 in, 2 out]
      n181 = property class="Arr (strict)"(reference=w209, "Value"=w208) -> ()  [unwired: 1 in, 2 out]
      n182 = property class="Bool (strict)"(reference=w206, "Value"=w203) -> ()  [unwired: 1 in, 2 out]
      n183 = property class="Arr (strict)"(reference=w205, "Value"=w202) -> ()  [unwired: 1 in, 2 out]
      n184 = property class="Clust (strict)"(reference=w204, "Value"=w201) -> ()  [unwired: 1 in, 2 out]
      n185 = To Unsigned Word Integer(number=w261) -> (unsigned 16bit integer=w260:u16)
      n186 = property class="DAQmxName"(reference=w238, "Value"=w233) -> ()  [unwired: 1 in, 2 out]
      n187 = property class="DAQmxName"(reference=w237, "Value"=w232) -> ()  [unwired: 1 in, 2 out]
      n188 = property class="DAQmxName"(reference=w236, "Value"=w231) -> ()  [unwired: 1 in, 2 out]
      n189 = property class="DAQmxName"(reference=w235, "Value"=w230) -> ()  [unwired: 1 in, 2 out]
      n190 = property class="DAQmxName"(reference=w234, "Value"=w229) -> ()  [unwired: 1 in, 2 out]
      n191 = property class="Clust (strict)"(reference=w259, "Value"=w258) -> ()  [unwired: 1 in, 2 out]
      n192 = property class="Clust (strict)"(reference=w220, "Value"=w219) -> ()  [unwired: 1 in, 2 out]
      n193 = property class="Clust (strict)"(reference=w165, "Value"=w164) -> ()  [unwired: 1 in, 2 out]
      n194 = call "Sys config window-Set wavelengths ring.vi"("Laser wavelength (nm)"=w260, "System Config window refs"=w187) -> ()  [unwired: 9 in, 1 out]
      n195 = property class="Clust (strict)"(reference=w269, "Value"=w166) -> ()  [unwired: 1 in, 2 out]
      n196 = property class="Bool (strict)"(reference=w228, "Value"=w226) -> ()  [unwired: 1 in, 2 out]
      n197 = property class="Clust (strict)"(reference=w227, "Value"=w225) -> ()  [unwired: 1 in, 2 out]
      n198 = property class="Bool (strict)"(reference=w188, "Value"=w186) -> ()  [unwired: 1 in, 2 out]
      n199 = property class="Enum (strict)"(reference=w250, "Value"=w212) -> ()  [unwired: 1 in, 2 out]
      n200 = property class="Bool (strict)"(reference=w249, "Value"=w246) -> ()  [unwired: 1 in, 2 out]
      n201 = property class="DigNum (strict)"(reference=w248, "Value"=w244) -> ()  [unwired: 1 in, 2 out]
      n202 = property class="Str"(reference=w247, "Value"=w243) -> ()  [unwired: 1 in, 2 out]
      n203 = property class="Clust (strict)"(reference=w241, "Value"=w239) -> ()  [unwired: 1 in, 2 out]
      n204 = property class="Clust (strict)"(reference=w222, "Value"=w221) -> ()  [unwired: 1 in, 2 out]
      n205 = property class="Bool (strict)"(reference=w190, "Value"=w189) -> ()  [unwired: 1 in, 2 out]
      n206 = property class="Bool (strict)"(reference=w242, "Value"=w240) -> ()  [unwired: 1 in, 2 out]
      n207 = property class="Bool (strict)"(reference=w197, "Value"=w199) -> ()  [unwired: 1 in, 2 out]
      n208 = property class="Clust (strict)"(reference=w198, "Value"=w200) -> ()  [unwired: 1 in, 2 out]
      n209 = property class="Clust (strict)"(reference=w224, "Value"=w223) -> ()  [unwired: 1 in, 2 out]
      n210 = property class="Bool (strict)"(reference=w196, "Value"=w195) -> ()  [unwired: 1 in, 2 out]
      n211 = property class="Bool (strict)"(reference=w194, "Value"=w193) -> ()  [unwired: 1 in, 2 out]
      n212 = property class="Clust (strict)"(reference=w217, "Value"=w218) -> ()  [unwired: 1 in, 2 out]
      n213 = property class="Bool (strict)"(reference=w192, "Value"=w191) -> ()  [unwired: 1 in, 2 out]
      n214 = property class="Clust (strict)"(reference=w277, "Value"=w275) -> ()  [unwired: 1 in, 2 out]
      n215 = property class="Clust (strict)"(reference=w276, "Value"=w161) -> ()  [unwired: 1 in, 2 out]
      n216 = property class="Clust (strict)"(reference=w163, "Value"=w159) -> ()  [unwired: 1 in, 2 out]
      n217 = property class="Str"(reference=w257, "Value"=w179) -> ()  [unwired: 1 in, 2 out]
      n218 = property class="Str"(reference=w256, "Value"=w178) -> ()  [unwired: 1 in, 2 out]
      n219 = property class="Str"(reference=w255, "Value"=w177) -> ()  [unwired: 1 in, 2 out]
      n220 = property class="Bool (strict)"(reference=w254, "Value"=w176) -> ()  [unwired: 1 in, 2 out]
      n221 = property class="DigNum (strict)"(reference=w253, "Value"=w175) -> ()  [unwired: 1 in, 2 out]
      n222 = property class="DigNum (strict)"(reference=w252, "Value"=w174) -> ()  [unwired: 1 in, 2 out]
      n223 = property class="DigNum (strict)"(reference=w251, "Value"=w173) -> ()  [unwired: 1 in, 2 out]
      n224 = property class="DigNum (strict)"(reference=w185, "Value"=w172) -> ()  [unwired: 1 in, 2 out]
      n225 = property class="DigNum (strict)"(reference=w184, "Value"=w171) -> ()  [unwired: 1 in, 2 out]
      n226 = property class="Bool (strict)"(reference=w183, "Value"=w170) -> ()  [unwired: 1 in, 2 out]
      n227 = property class="Bool (strict)"(reference=w182, "Value"=w169) -> ()  [unwired: 1 in, 2 out]
      n228 = Bundle By Name(cluster=T29 {"Microscope ID"="003", "Microscope Type"="AOLM", "Revision Number"="1.0.0.0", "Advanced Imaging"=FALSE, "Error Logging"=FALSE, "Performance Monitoring"=FALSE, "Max Allowed Trial Length"=60.0, "Initial Scan Resolution"=512.0, "Initial Acceptance Angle"=5.0, "Initial Laser Wavelength"=900.0, "Initial Dwell Time"=900.0} ("Cluster"), "Microscope ID"=w179, "Microscope Type"=w178, "Revision Number"=w177, "Advanced Imaging"=w176, "Max Allowed Trial Length"=w175, "Initial Scan Resolution"=w174, "Initial Acceptance Angle"=w173, "Initial Laser Wavelength"=w172, "Initial Dwell Time"=w171, "Error Logging"=w170, "Performance Monitoring"=w169) -> (w168:T29)
    }
  }
  "error out" <- w19
  n229 = Bundle By Name(cluster=T1 {"Triggers output setup"=[], "General trigger settings"={"Trigger 1 function"=enum."Encoder trigger", "Triggers loop clock (MHz)"=0.0}, "Calibration settings"={"Pockels cal.Zoom"=0, "Pockels cal.Dwell time (µs)"=0.0}, "Hardware Configuration"={"Dev. PC"=FALSE, "Swap XY on stage"=FALSE, "No of AOD"=0, "Computer MAC address"="", "Externalise Triggers"=FALSE, "Trigger HW config"={"Available Device List"=0, "Device Address"=""}, "DAQmx Chan"={"Pockels AO"="", "Hard shutter AO"="", "PMT AOs"="", "Galvo AOs"="", "Power meter AI"=""}, "XY stage available"=FALSE, "XY Stage"={"COM port"="", "Baudrate"=0, "Type"=""}, "Z stage available"=FALSE, "Z Stage config cluster"={"COM port"="", "Baudrate"=0, "Type"=""}, "Encoder available"=FALSE, "Encoder"={"IP address"="", "Port"=0, "Wheel radius (cm)"=0.0, "Encoder Trigger"=""}, "VidRec available"=FALSE, "Cam VidRec"={"DO flag-Video record"="", "DO flag-Trial start"=""}, "Laser Power Control HW config"={"Laser Power Control"="", "Laser Power Modulation Control"=enum."NI"}, "Laser 1 available"=FALSE, "Laser 1 config cluster"={"COM port"="", "Baud Rate"=0, "Type"=""}, "Prechirper 1 available"=FALSE, "Prechirper 1 config cluster"={"Type"="", "Baud Rate"=0, "COM port"=""}, "Control system.FPGA available?"=FALSE, "Control Sys. HW config"={"Control system.FPGA Type"=enum."Virtex 5", "Control system.Network adapter name"="", "Control system.MAC address"="", "Control system.Ethernet Port"=0, "Control system.Ethernet Port Opened"=FALSE}, "DAQ FPGA HW Config"={"FGPA Ref"=refnum, "Target"="", "input card type"=enum."AC Card"}}, "System Config"={"Laser wavelength (nm)"=0.0, "DAQ FPGA System"={"Clock Freq (MHz) "=0.0, "Samples Wait after Trigger"=0, "AOD fill"=0, "StartupDelay"=0, "Slip Cycle (clock cycles)"=0, "Add Cycle"=FALSE}, "Control system"={"AOD 1 Amplitude"=0, "AOD 2 Amplitude"=0, "AOD 3 Amplitude"=0, "AOD 4 Amplitude"=0, "AOD 5 Amplitude"=0, "AOD 6 Amplitude"=0, "T0 (ns)"=0.0, "Ta (ns)"=0.0, "Data Time Interval (ns)"=0.0, "Ctrl FPGA Clock (MHz)"=0.0}}, "Calibration config."={"Current Objective"="", "Objective Settings"=[], "PreChirper Values Preset ?"=FALSE, "PreChirper Settings"=[], "PreChirper Constants"={"a 1"=0, "b 1"=0, "c 1"=0, "a 2"=0, "b 2"=0, "c 2"=0, "lmin"=0, "lmax"=0}}, "General Setup"={"Microscope ID"="003", "Microscope Type"="AOLM", "Revision Number"="1.0.0.0", "Advanced Imaging"=FALSE, "Error Logging"=FALSE, "Performance Monitoring"=FALSE, "Max Allowed Trial Length"=60.0, "Initial Scan Resolution"=512.0, "Initial Acceptance Angle"=5.0, "Initial Laser Wavelength"=900.0, "Initial Dwell Time"=900.0}, "AOD Settings - distilled"={"AOD 1 thickness (mm)"=0.0, "AOD 2 thickness (mm)"=0.0, "AOD 3 thickness (mm)"=0.0, "AOD 4 thickness (mm)"=0.0, "AOD 1-2 separation (mm)"=0.0, "AOD 2-3 separation (mm)"=0.0, "AOD 3-4 separation (mm)"=0.0, "AOD 1 Centre (mm)"=0.0, "AOD 2 Centre (mm)"=0.0, "AOD 3 Centre (mm)"=0.0, "AOD 4 Centre (mm)"=0.0, "AOD 1 X Offset"=0.0, "AOD 2 X Offset"=0.0, "AOD 3 X Offset"=0.0, "AOD 4 X Offset"=0.0, "AOD 1 Y Offset"=0.0, "AOD 2 Y Offset"=0.0, "AOD 3 Y Offset"=0.0, "AOD 4 Y Offset"=0.0, "Timing Offset AOD 1"=0.0, "Timing Offset AOD 2"=0.0, "Timing Offset AOD 3"=0.0, "Timing Offset AOD 4"=0.0, "AOL centre wavelength (nm)"=0.0, "AOL centre frequency (MHz)"=0.0, "Pair deflection ratio"=0.0, "AOL aperture (mm)"=0.0, "AOD fill time (us)"=0.0, "Diffraction mode"=0.0, "Crystal length (mm)"=0.0, "Acoustic velocity (m/s)"=0.0, "AOD Ord. Refractive index"=0.0}} ("Initial configuration"), "General Setup"=w3, "Hardware Configuration"=w6, "System Config"=w5, "Triggers output setup"=w18, "General trigger settings"=w14, "AOD Settings - distilled"=w2, "Calibration settings"=w15, "Calibration config."=w4) -> (→"output cluster":T1)
